vi "BalanceRudderSailSuggestion.vi"(11 "ForceOnRudder":dbl) -> (3 "SailSuggestion":dbl)   [LabVIEW 2012]
doc: "Takes in some measure of weather helm. This may be force on rudder, position of rudder (not straight when it should be straight), or even ate of turn when we should be going straight. The algorithm then decides how to adjust the sails to balance that weather helm."
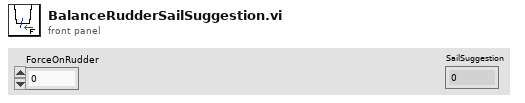
[diagram p1: front panel]
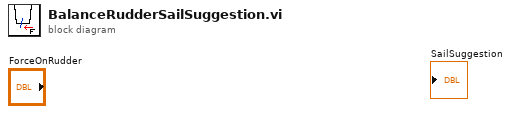
[diagram p0: block diagram]
diagram:
